vi "changeFileExtension.vi"(9 "extension":string, 10 "Path":path) -> (2 "Path out":path)   [LabVIEW 2009, in "Tools.lvlib" / "Filing.lvlib"]
uses:
  Filing.lvlib
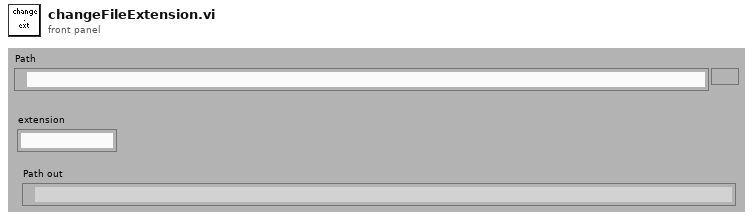
[diagram p1: front panel]
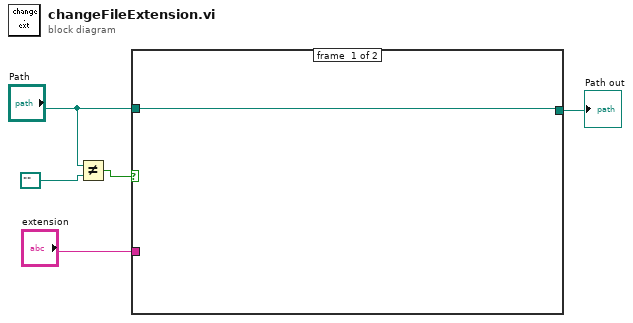
[diagram p0: block diagram]
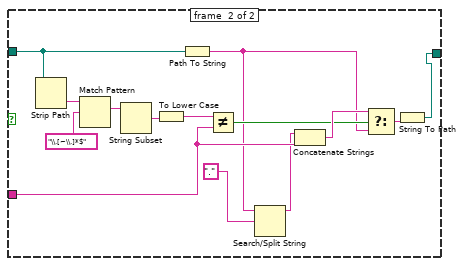
[diagram p2: hidden frame]
diagram:
  n1 = Not Equal?(x="Path", y=path "") -> (x != y?=w1:bool)
  n2 = case shown="True" w1 {
    tunnel: [w6 w20] -> w5
    tunnel: "Path" -> [w6 w11]
    tunnel: "extension" -> [_ w10]
    frame #0 {
    }
    frame #1 {
      n3 = Strip Path(path=w11) -> (name=w16:string)  [unwired: 1 out]
      n4 = Match Pattern(string=w16, regular expression="\\.[~\\.]*$") -> (match substring=w17:string)  [unwired: 1 in, 3 out]
      n5 = String Subset(string=w17) -> (substring=w15:string)  [unwired: 2 in]
      n6 = To Lower Case(string=w15) -> (all lower case string=w13:string)
      n7 = Path To String(path=w11) -> (string=w9:string)
      n8 = Not Equal?(x=w13, y=w10) -> (x != y?=w12:bool)
      n9 = Search/Split String(string=w9, search string/char (-)=".") -> (substring before match=w7:string)  [unwired: 1 in, 2 out]
      n10 = Concatenate Strings(w7, w10) -> (w19:string)
      n11 = Select(t=w19, s=w12, f=w9) -> (s? t:f=w18:string)
      n12 = String To Path(string=w18) -> (path=w20:path)
    }
  }
  "Path out" <- w5
